vi "FinalSteering.vi"() -> ()   [LabVIEW 2015]
uses:
  GlobalPath.vi
  GlobalVi.vi
  GlobalData.vi
panel:
  out "ChoosePanel":bool
  in  "Choose Panel":bool
  out "Lines":string[](array[string])
  out "GlueSideUp":bool
  out "GlueSideDown":bool
  in  "Stuccatture side up":bool
  in  "Stuccatture/Washer side down":bool
  in  "current vi path":path
  out "Opening program":string
  in  "HV filters, grounding and cabling":bool
  out "HV":bool
  # "Status"
  # "Control"
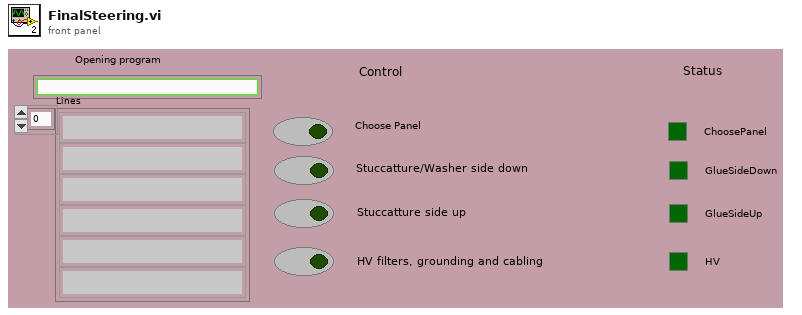
[diagram p1: front panel]
types:
  T1 = enum16{"open", "replace", "create", "open or create", "replace or create", "replace or create with confirmation"}
  T2 = enum32{"Bad", "Idle", "Run top level", "Running"}
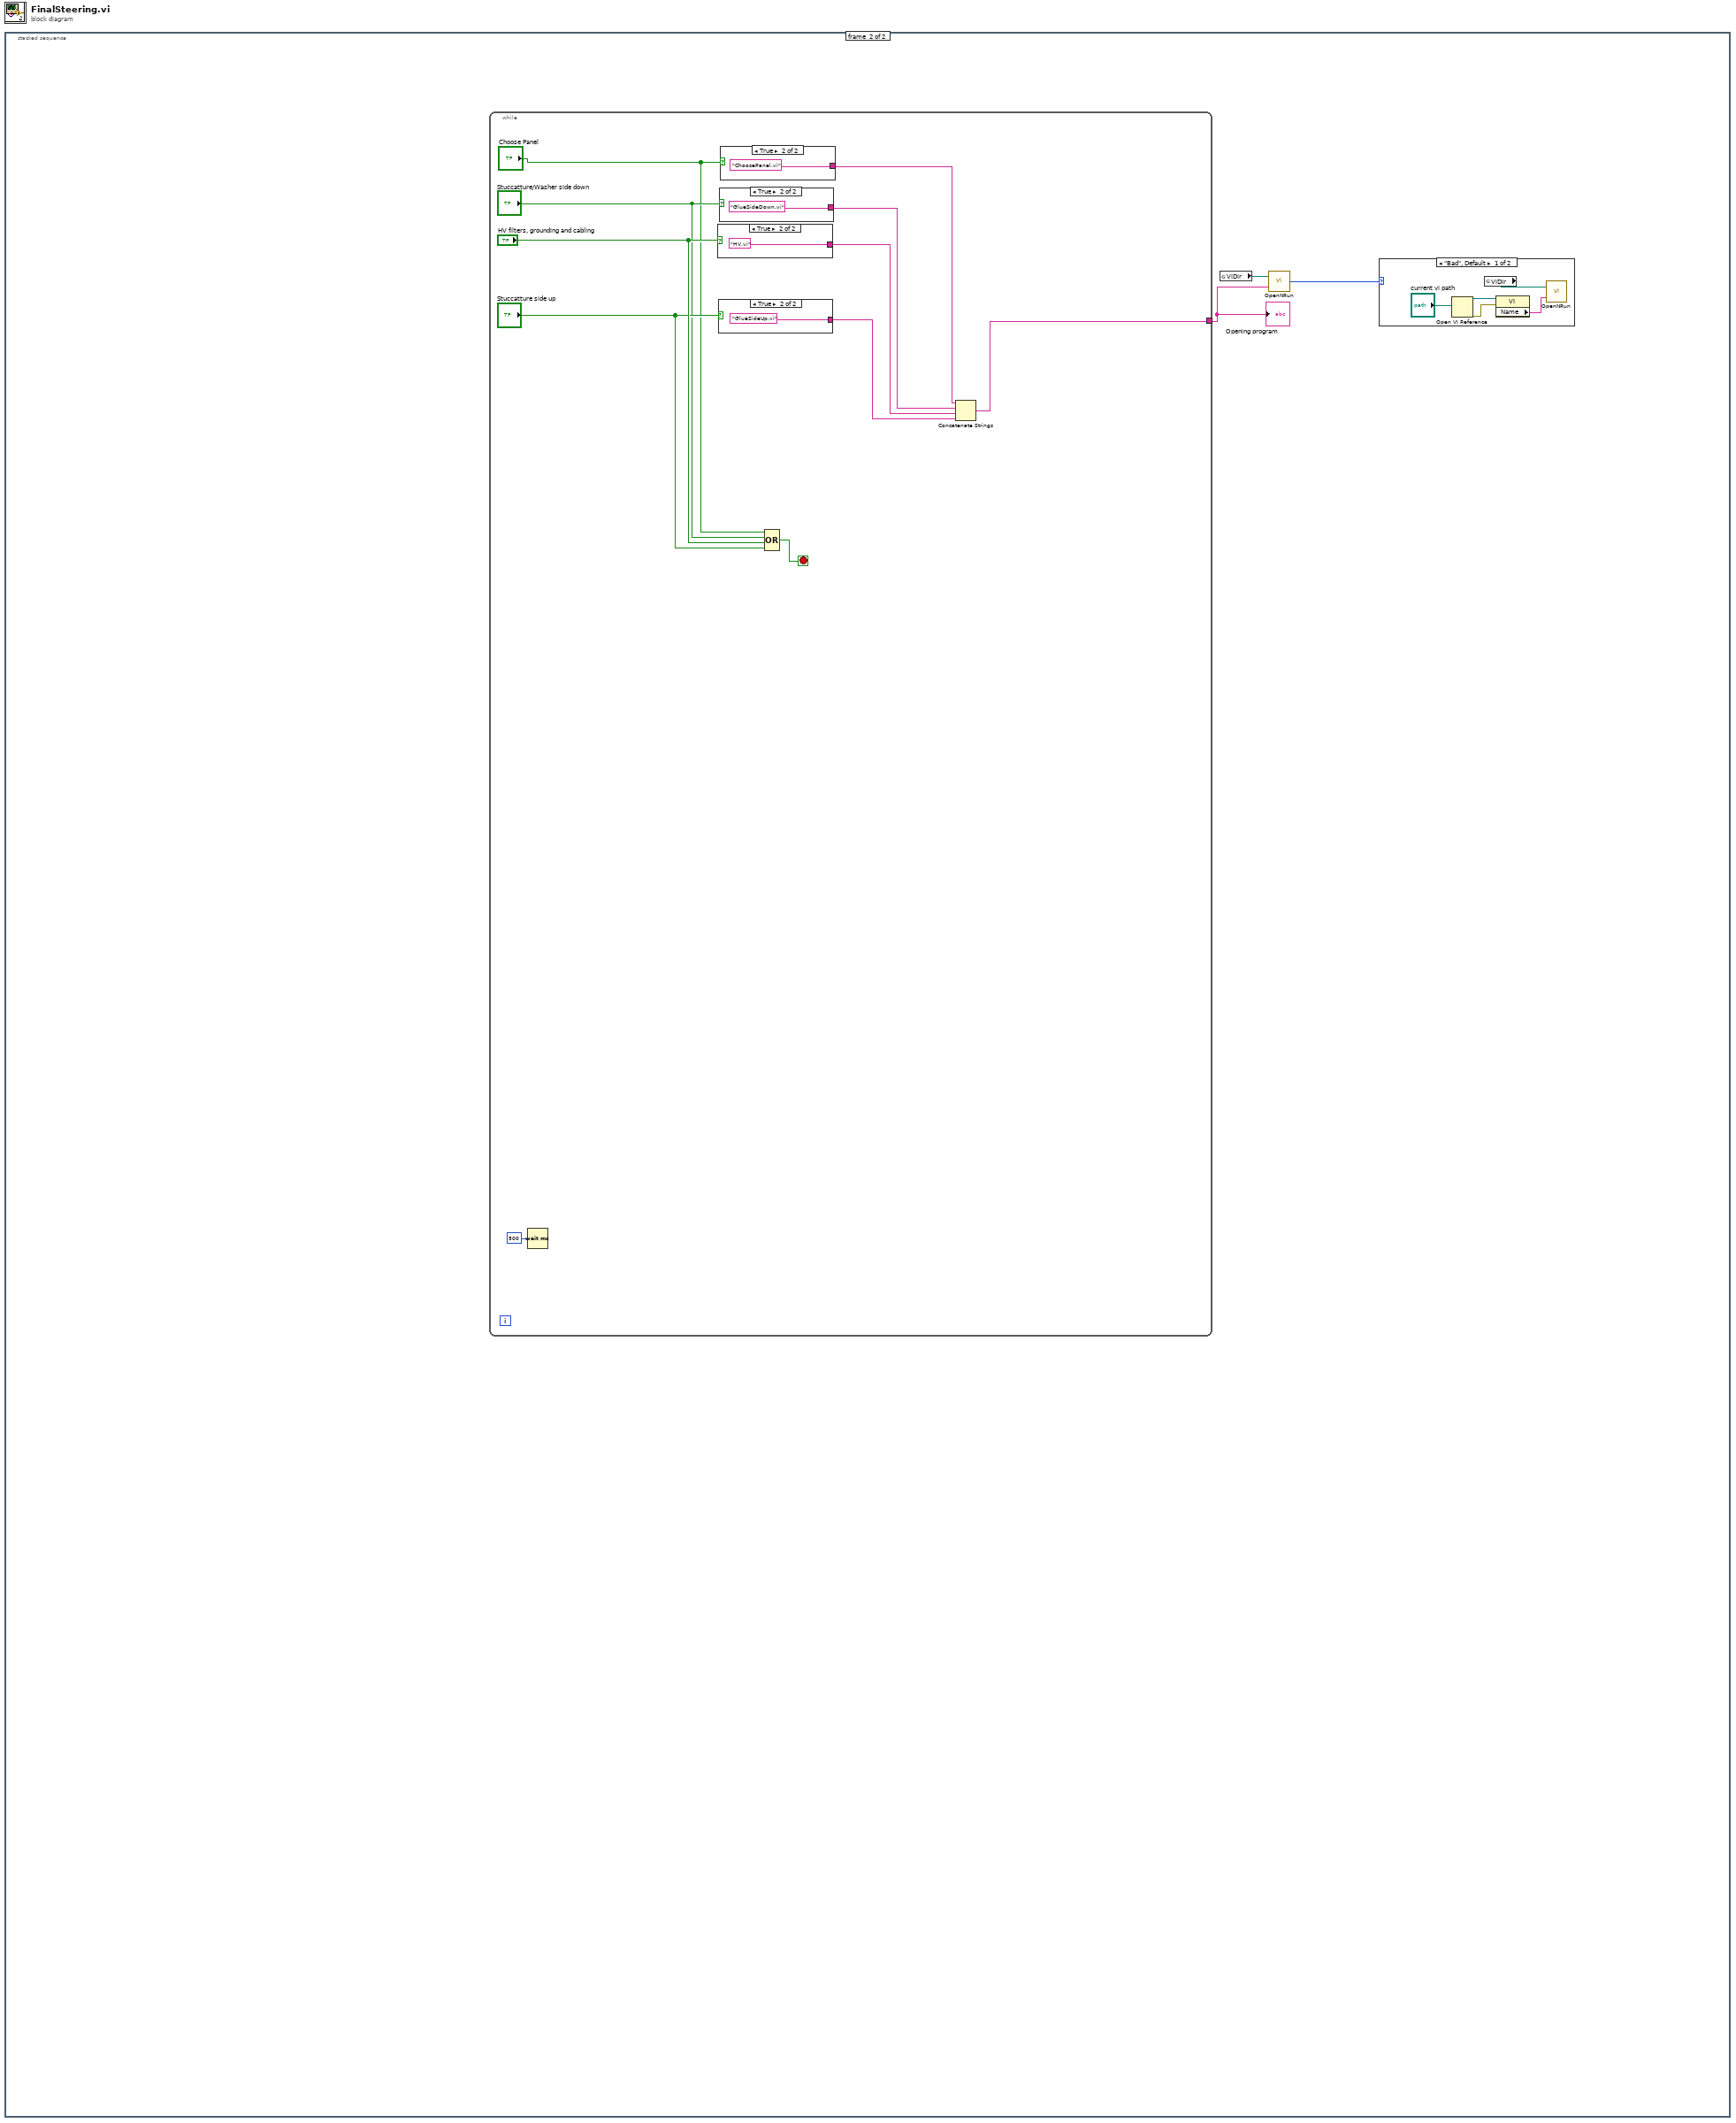
[diagram p0: block diagram]
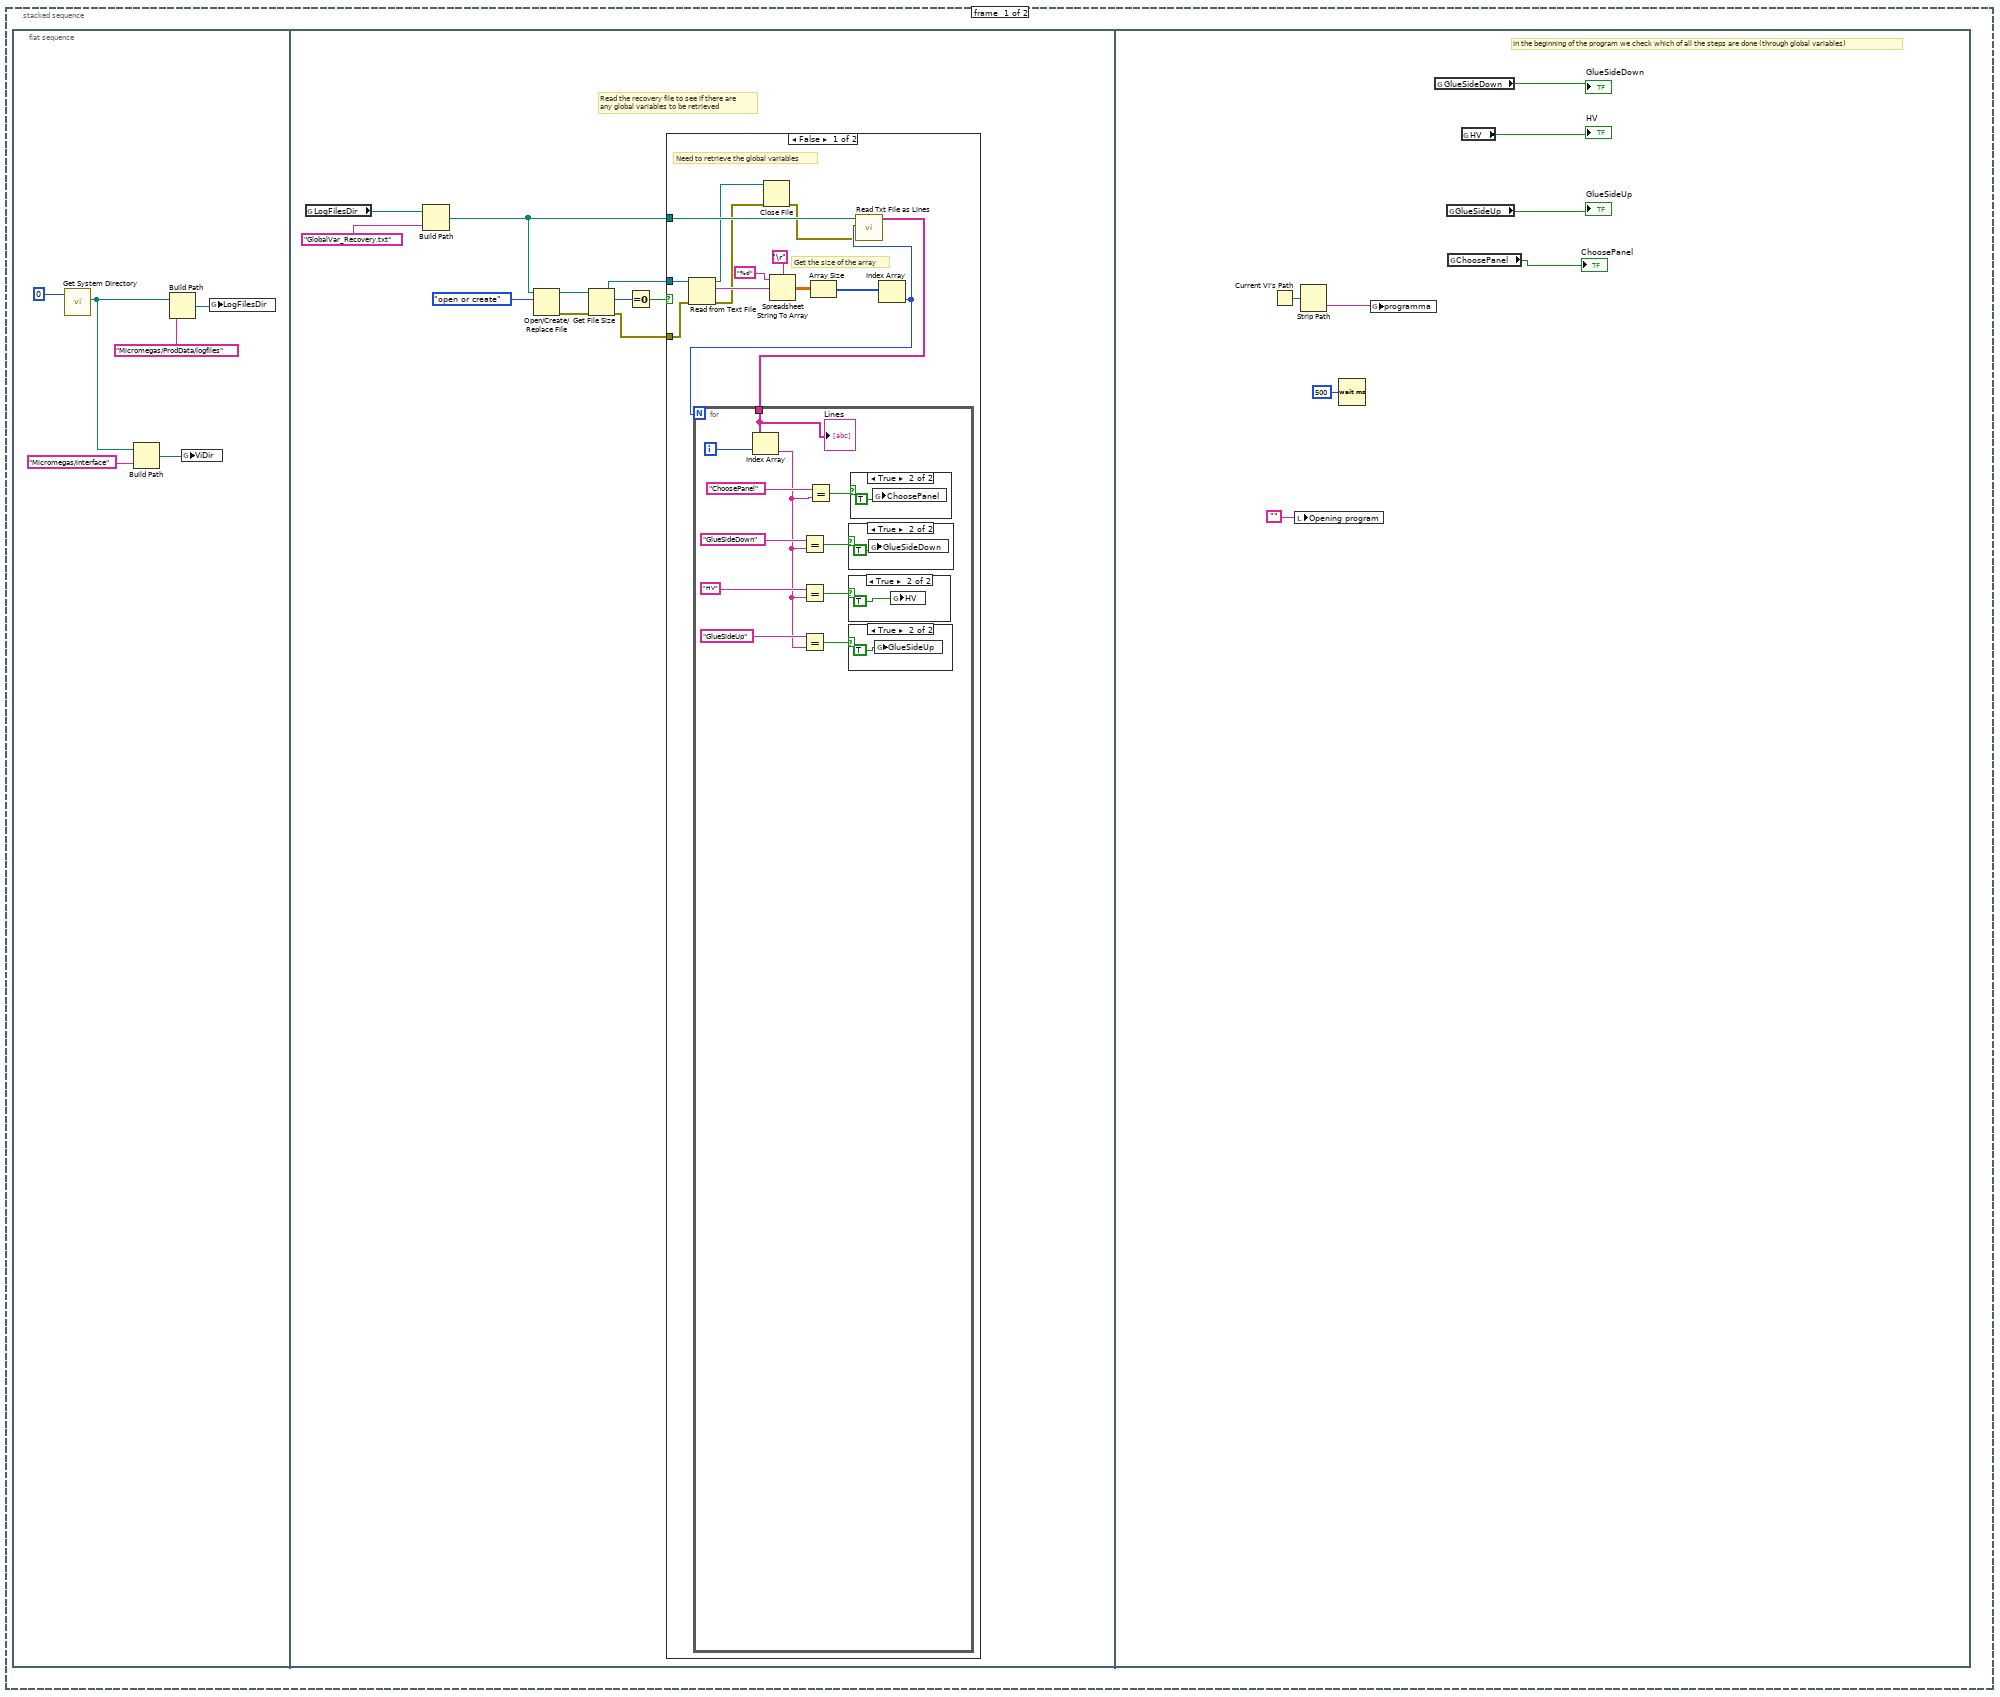
[diagram p2: hidden frame]
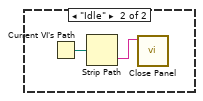
[diagram p8: hidden frame]
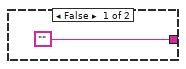
[diagram p9: hidden frame]
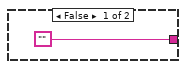
[diagram p10: hidden frame]
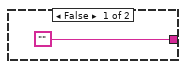
[diagram p11: hidden frame]
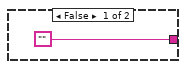
[diagram p12: hidden frame]
diagram:
  n1 = stacked-sequence {
    frame #0 {
      n2 = flat-sequence {
        frame #0 {
          n3 = call <vilib>:"Get System Directory.vi"("system directory type"=0) -> ("system directory"=w4:path)  [unwired: 10 in]
          n4 = Build Path(base path=w4, name or relative path="Micromegas/interface") -> (appended path=w3:path)
          n5 = Build Path(base path=w4, name or relative path="Micromegas/ProdData/logfiles") -> (appended path=w1:path)
          n6 = global write "GlobalPath.vi" "ViDir"(w3) -> ()
          n7 = global write "GlobalPath.vi" "LogFilesDir"(w1) -> ()
        }
        frame #1 {
          # "Read the recovery file to see if there are\nany global variables to be retrieved"
          n8 = global read "GlobalPath.vi" "LogFilesDir"() -> (w7:path)
          n9 = Build Path(base path=w7, name or relative path="GlobalVar_Recovery.txt") -> (appended path=w8:path)
          n10 = Open/Create/Replace File(file path (use dialog)=w8, operation (0:open)=T1."open or create") -> (refnum out=w15:refnum<file>, error out=w13:errorcluster)  [unwired: 4 in, 1 out]
          n11 = Get File Size(file=w15, error in=w13) -> (refnum out=w11:refnum<file>, size (in bytes)=w14:i64, 0:w10:errorcluster)
          n12 = Equal To 0?(x=w14) -> (x = 0?=w12:bool)
          n13 = case shown="False" w12 {
            tunnel: w11 -> [w24 _]
            tunnel: w10 -> [w26 _]
            tunnel: w8 -> [w23 _]
            frame False {
              # "Get the size of the array"
              # "Need to retrieve the global variables"
              n14 = Read from Text File(file (use dialog)=w24, error in=w26) -> (refnum out=w19:refnum<file>, text=w27:string, error out=w18:errorcluster)  [unwired: 3 out]
              n15 = Close File(refnum=w19, error in=w18) -> (error out=w17:errorcluster)  [unwired: 1 out]
              n16 = Spreadsheet String To Array(delimiter (Tab)="\r", format string="%d", spreadsheet string=w27) -> (array=w25:dbl[][])  [unwired: 1 out]
              n17 = Array Size(array=w25) -> (size(s)=w22:i32[])
              n18 = Index Array(array=w22) -> (element=w20:i32)  [unwired: 1 in]
              n19 = call "Read Txt File as Lines.vi"("error in"=w17, "Lines to Read"=w20, "file path (use dialog)"=w23) -> ("Lines"=w21:string[])  [unwired: 7 in, 1 out]
              n20 = for {
                N: w20 -> [_]
                tunnel: w21 -> [w33]
                i -> [w34]
                n21 = Index Array(array=w33, index=w34) -> (element=w31:string)
                n22 = Equal?(x="GlueSideDown", y=w31) -> (x = y?=w40:bool)
                n23 = Equal?(x="HV", y=w31) -> (x = y?=w39:bool)
                n24 = Equal?(x="GlueSideUp", y=w31) -> (x = y?=w38:bool)
                n25 = Equal?(x="ChoosePanel", y=w31) -> (x = y?=w30:bool)
                n26 = case shown="True" w40 {
                  frame False {
                  }
                  frame True {
                    n27 = global write "GlobalVi.vi" "GlueSideDown"(TRUE) -> ()
                  }
                }
                n28 = case shown="True" w39 {
                  frame False {
                  }
                  frame True {
                    n29 = global write "GlobalVi.vi" "HV"(TRUE) -> ()
                  }
                }
                n30 = case shown="True" w38 {
                  frame False {
                  }
                  frame True {
                    n31 = global write "GlobalVi.vi" "GlueSideUp"(TRUE) -> ()
                  }
                }
                n32 = case shown="True" w30 {
                  frame False {
                  }
                  frame True {
                    n33 = global write "GlobalVi.vi" "ChoosePanel"(TRUE) -> ()
                  }
                }
                "Lines" <- w33
              }
            }
            frame True {
              # "File is empty so nothing to retrieve"
            }
          }
        }
        frame #2 {
          # "In the beginning of the program we check which of all the steps are done (through global variables)"
          n34 = Current VI's Path() -> (path=w52:path)
          n35 = local write "Opening program"("") -> ()
          n36 = Strip Path(path=w52) -> (name=w48:string)  [unwired: 1 out]
          n37 = Wait (ms)(milliseconds to wait=u32 500) -> ()  [unwired: 1 out]
          n38 = global write "GlobalData.vi" "programma"(w48) -> ()
          n39 = global read "GlobalVi.vi" "GlueSideDown"() -> (→"GlueSideDown":bool)
          n40 = global read "GlobalVi.vi" "GlueSideUp"() -> (→"GlueSideUp":bool)
          n41 = global read "GlobalVi.vi" "ChoosePanel"() -> (→"ChoosePanel":bool)
          n42 = global read "GlobalVi.vi" "HV"() -> (→"HV":bool)
        }
      }
    }
    frame #1 {
      n43 = while {
        tunnel: [w71] -> w55
        stop <- w72 stop-if-true
        n44 = Wait (ms)(milliseconds to wait=u32 500) -> ()  [unwired: 1 out]
        n45 = case shown="True" "HV filters, grounding and cabling" {
          tunnel: ["" "HV.vi"] -> w70
          frame False {
          }
          frame True {
          }
        }
        n46 = case shown="True" "Stuccatture side up" {
          tunnel: ["" "GlueSideUp.vi"] -> w68
          frame False {
          }
          frame True {
          }
        }
        n47 = case shown="True" "Stuccatture/Washer side down" {
          tunnel: ["" "GlueSideDown.vi"] -> w69
          frame False {
          }
          frame True {
          }
        }
        n48 = case shown="True" "Choose Panel" {
          tunnel: ["" "ChoosePanel.vi"] -> w64
          frame False {
          }
          frame True {
          }
        }
        n49 = Compound Arithmetic op=OR("Choose Panel", "Stuccatture/Washer side down", "HV filters, grounding and cabling", "Stuccatture side up") -> (w72:bool)
        n50 = Concatenate Strings(w64, w69, w70, w68) -> (w71:string)
      }
      "Opening program" <- w55
      n51 = global read "GlobalPath.vi" "ViDir"() -> (w53:path)
      n52 = call "OpenNRun.vi"("VI name"=w55, "ViDirPath"=w53) -> ("Execution:State"=w54:T2)
      n53 = case shown="\"Bad\", Default" w54 {
        frame "Bad", Default {
          n54 = Open VI Reference(vi path="current vi path") -> (vi reference=w60:refnum<vi>, error out=w59:errorcluster)  [unwired: 5 in]
          n55 = global read "GlobalPath.vi" "ViDir"() -> (w57:path)
          n56 = property class="VI"(reference=w60, error in=w59) -> ("Name"=w56:string)  [unwired: 2 out]
          n57 = call "OpenNRun.vi"("VI name"=w56, "ViDirPath"=w57) -> ()  [unwired: 1 out]
        }
        frame "Idle" {
          n58 = Current VI's Path() -> (path=w61:path)
          n59 = Strip Path(path=w61) -> (name=w62:string)  [unwired: 1 out]
          n60 = call <vilib>:"Close Panel.vi"("VI name"=w62) -> ()  [unwired: 10 in, 1 out]
        }
      }
    }
  }
